vi "Fake Digital out.vi"(8 "error in (no error)":errorcluster, 10 "Value to DO":bool, 11 "DO select":dbl) -> (0 "error out":errorcluster)   [LabVIEW 2013]
panel:
  out "indicator":bool
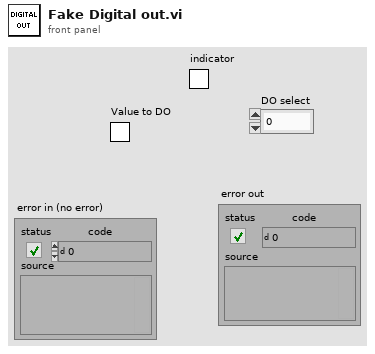
[diagram p1: front panel]
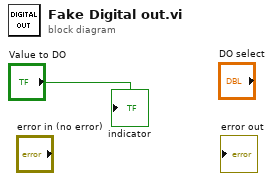
[diagram p0: block diagram]
diagram:
  "indicator" <- "Value to DO"
